vi "Alphabetize Case-Sensitive Cluster Constant.vi"(8 "Error In":errorcluster) -> (0 "Error Out":errorcluster)   [LabVIEW 2017, in "Tests.lvlib" / "Toolkit.lvlib"]
uses:
  Toolkit.lvlib
  <vilib>/Utility/traverseref.llb/TRef TravTarget.ctl
  Support/Alphabetize Case-Sensitive Cluster Constant Target.vi
  <vilib>/addons/_JKI Toolkits/Caraya/classes/Test/Test.lvclass
  src/Toolkit/Toolkit.lvlib
  <vilib>/Utility/traverseref.llb/VI Scripting - Traverse.lvlib
  <vilib>/addons/_JKI Toolkits/Caraya/classes/Assert/Assert.lvclass
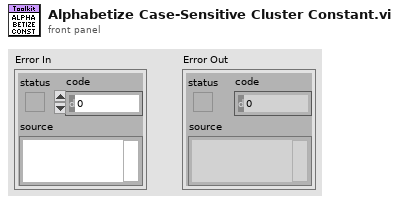
[diagram p1: front panel]
types:
  T1 = typedef "TRef TravTarget.ctl" = enum16{"FP", "BD", "Other"}
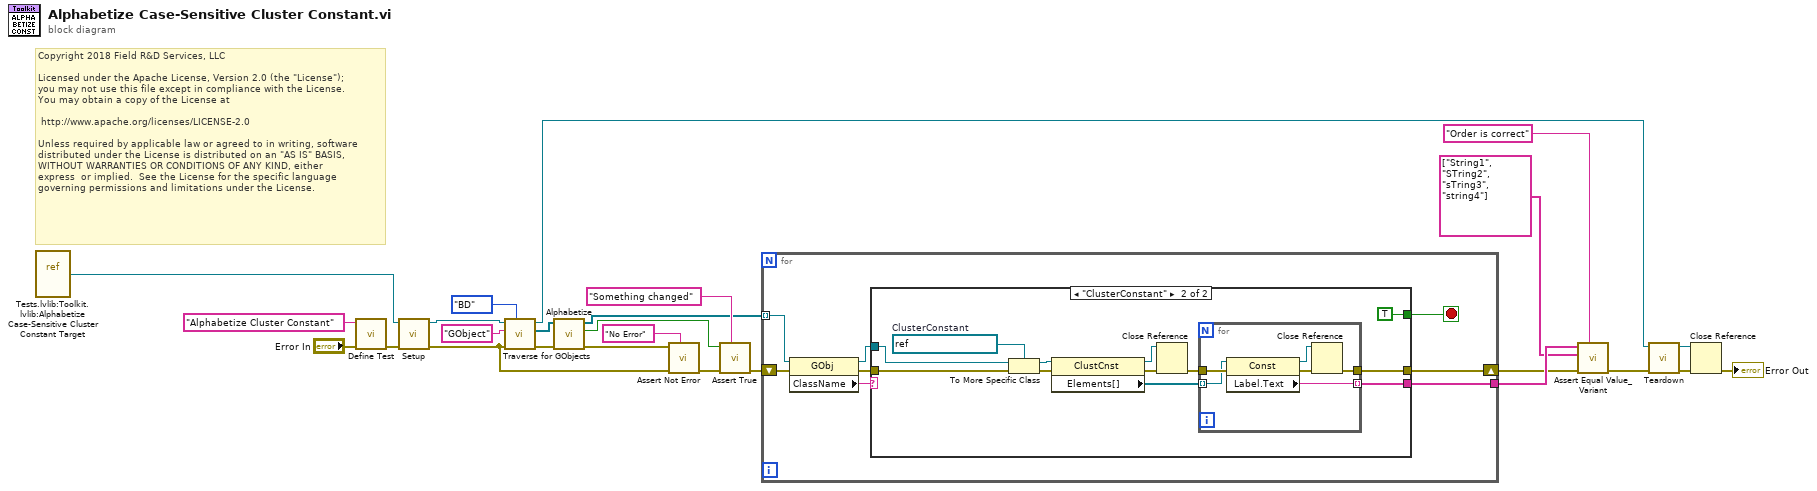
[diagram p0: block diagram]
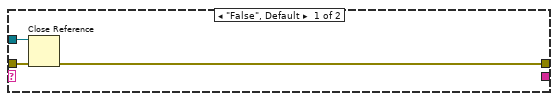
[diagram p2: hidden frame]
diagram:
  # "Copyright 2018 Field R&D Services, LLC\n\nLicensed under the Apache License, Version 2.0 (the \"License\");\nyou may not use this file except in compliance with the License.\nYou may obtain a copy of the License at\n\n\thttp://www.apache.org/licenses/LICENSE-2.0\n\nUnless required by applicable law or agreed to in writing, software\ndistributed under the License is distributed on an \"AS IS\" BASIS,\nWITHOUT WARRANTIES OR CONDITIONS OF ANY KIND, either \nexpress  or implied.  See the License for the specific language \ngoverning permissions and limitations under the License."
  n1 = vi-ref "Tests.lvlib:Toolkit.lvlib:Alphabetize Case-Sensitive Cluster Constant Target.vi"() -> (w23:refnum<vi>)
  n2 = call <vilib>:"Define Test.vi"("error in (no error)"="Error In", "Label (VI Title)"="Alphabetize Cluster Constant") -> ("error out"=w24:errorcluster)  [unwired: 9 in]
  n3 = call "Setup.vi"("Error In"=w24, "VI In"=w23) -> ("Error Out"=w13:errorcluster, "VI Out"=w21:refnum<vi>)  [unwired: 8 in]
  n4 = call <vilib>:"Traverse for GObjects.vi"("Traverse Target"=TRef_TravTarget."BD", "error in (no error)"=w13, "Class Name"="GObject", "VI Refnum"=w21) -> ("error out"=w7:errorcluster, "References"=w6:refnum<vi>[], "dup VI Refnum"=w11:refnum<vi>)  [unwired: 4 in, 1 out]
  n5 = call "Alphabetize.vi"("Error In"=w7, "Clusters In"=w6) -> ("Error Out"=w16:errorcluster, "Change?"=w4:bool, "Clusters Out"=w2:refnum<vi>[])  [unwired: 7 in]
  n6 = call <vilib>:"Assert Not Error.vi"("Label"="No Error", "error in (no error)"=w13, "Not Error?"=w16) -> ("error out"=w15:errorcluster)  [unwired: 8 in]
  n7 = call <vilib>:"Assert True.vi"("Label"="Something changed", "error in (no error)"=w15, "True?"=w4) -> ("error out"=w5:errorcluster)  [unwired: 8 in]
  n8 = for {
    tunnel: [w34] -> w19
    shift-right: [w33] -> w14
    shift-left: w5 -> [w32]
    tunnel: w2 -> [w30] mode=indexing
    stop <- w27 stop-if-true
    n9 = property class="GObj"(reference=w30, error in=w32) -> (reference out=w28:refnum<vi>, error out=w31:errorcluster, "ClassName"=w29:string)
    n10 = case shown="\"ClusterConstant\"" w29 {
      tunnel: [_ w45] -> w34
      tunnel: [w36 w44] -> w33
      tunnel: w31 -> [w37 w40]
      tunnel: w28 -> [w35 w39]
      tunnel: [_ TRUE] -> w27
      frame "False", Default {
        n11 = Close Reference(reference=w35, error in (no error)=w37) -> (error out=w36:errorcluster)
      }
      frame "ClusterConstant" {
        w41 = refnum<vi> refnum  # ClusterConstant
        n12 = To More Specific Class(target class=w41, reference=w39, error in=w40) -> (specific class reference=w42:refnum<vi>, error out=w43:errorcluster)
        n13 = property class="ClustCnst"(reference=w42, error in=w43) -> (reference out=w46:refnum<vi>, error out=w48:errorcluster, "Elements[]"=w49:refnum<vi>[])
        n14 = Close Reference(reference=w46, error in (no error)=w48) -> (error out=w47:errorcluster)
        n15 = for {
          tunnel: w49 -> [w50] mode=indexing
          tunnel: w47 -> [w55]
          tunnel: [w54] -> w45 mode=indexing
          tunnel: [w51] -> w44
          n16 = property class="Const"(reference=w50, error in=w55) -> (reference out=w52:refnum<vi>, error out=w53:errorcluster, "Label.Text"=w54:string)
          n17 = Close Reference(reference=w52, error in (no error)=w53) -> (error out=w51:errorcluster)
        }
      }
    }
  }
  n18 = call <vilib>:"Assert Equal Value_Variant.vi"("Label"="Order is correct", "error in (no error)"=w14, "Y"=string[] ["String1", "STring2", "sTring3", "string4"], "X"=w19) -> ("error out"=w12:errorcluster)  [unwired: 7 in]
  n19 = call "Teardown.vi"("Error In"=w12, "VI In"=w11) -> ("Error Out"=w9:errorcluster, "VI Out"=w10:refnum<vi>)  [unwired: 8 in]
  n20 = Close Reference(reference=w10, error in (no error)=w9) -> (error out=→"Error Out":errorcluster)
